vi "PartInfo_SM.vi"(8 "error in (no error)":errorcluster, 10 "PartInfo":T1, 11 "Inspection Statemachine in":refnum<class "Inspection Statemachine.lvclass">) -> (0 "error out":errorcluster, 3 "Inspection Statemachine out":refnum<class "Inspection Statemachine.lvclass">)   [LabVIEW 2019, in "Inspection Statemachine.lvclass"]
uses:
  Inspection Statemachine.lvclass
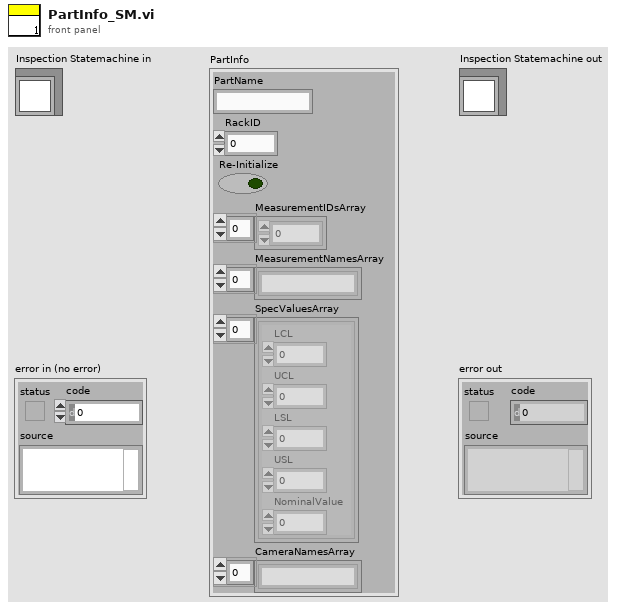
[diagram p1: front panel]
types:
  T1 = cluster{"PartName":string, "RackID":u8, "Re-Initialize":bool, "MeasurementIDsArray":u16[], "MeasurementNamesArray":string[], "SpecValuesArray":cluster{"LCL":dbl, "UCL":dbl, "LSL":dbl, "USL":dbl, "NominalValue":dbl}[], "CameraNamesArray":string[]}
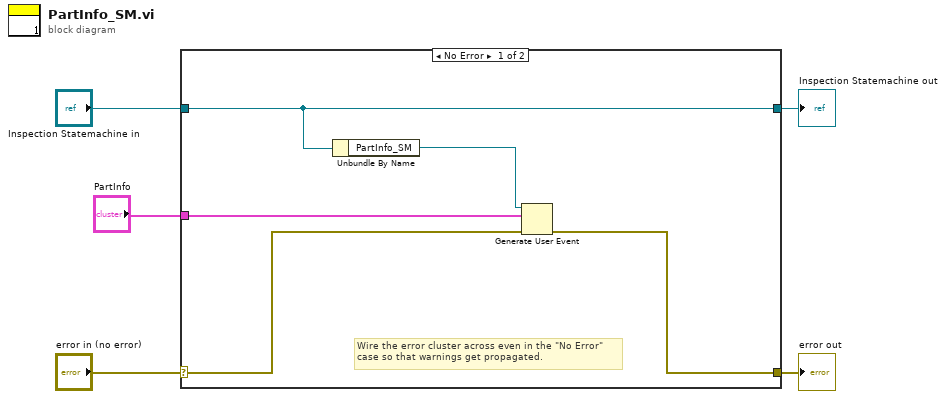
[diagram p0: block diagram]
diagram:
  n1 = case shown="No Error" "error in (no error)" {
    selector: "error in (no error)" -> [w7 w12]
    tunnel: [w6 w12] -> w4
    tunnel: [w10 w11] -> w2
    tunnel: "Inspection Statemachine in" -> [w10 w11]
    tunnel: "PartInfo" -> [w8 _]
    frame No Error {
      # "Wire the error cluster across even in the \"No Error\"\ncase so that warnings get propagated."
      n2 = Unbundle By Name(w10) -> ("PartInfo_SM"=w9:refnum<user-event>)
      n3 = Generate User Event(user event=w9, event data cluster=w8, error in=w7) -> (error out=w6:errorcluster)  [unwired: 1 in, 1 out]
    }
    frame Error {
    }
  }
  "error out" <- w4
  "Inspection Statemachine out" <- w2
